vi "DispenseOnOff_Boolean.vi"(10 "Value":bool=TRUE, 11 "I-O in":refnum<class "Copy of I-O.lvclass">) -> (3 "I-O out":refnum<class "Copy of I-O.lvclass">)   [LabVIEW 2016]
uses:
  Copy of I-O.lvclass
panel:
  out "error out":errorcluster
  in  "error in (no error)":errorcluster
  # "Dispense On/Off"
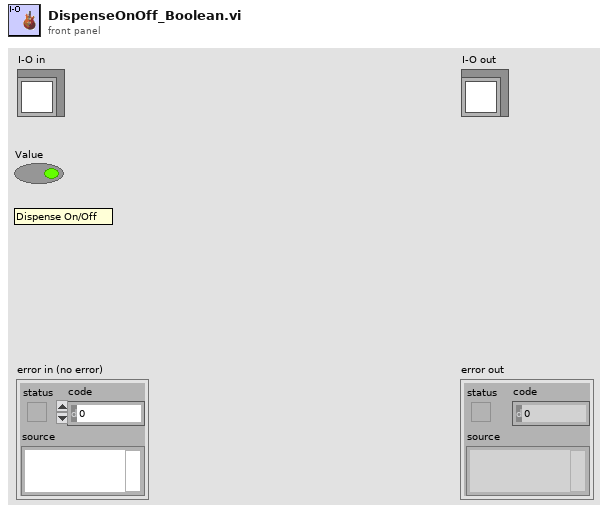
[diagram p1: front panel]
types:
  T1 = typedef "Copy of I-O.lvclass/Pin Map.ctl" = cluster{"Region Valves":i32[], "Extra Valves":dbl[][], "Tool Primary Valve":i32, "Tool Secondary Valve":i32, "Region Sensors":i32[], "Extra Sensors":dbl[][], "Tool Primary Sensor":dbl, "Tool Secondary Sensor":dbl, "Compression Sensor":dbl, "5V":i32, "NTU_Glue":dbl}
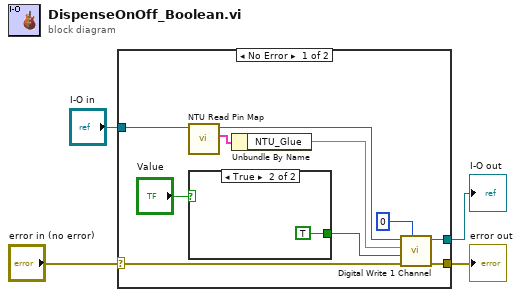
[diagram p0: block diagram]
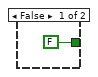
[diagram p2: hidden frame]
diagram:
  n1 = case shown="No Error" "error in (no error)" {
    selector: "error in (no error)" -> [w13 w18]
    tunnel: [w12 w18] -> w3
    tunnel: [w14 w17] -> w1
    tunnel: "I-O in" -> [w7 w17]
    frame No Error {
      n2 = call-dynamic "NTU Read Pin Map.vi"("I-O in"=w7) -> ("Pin Map"=w6:T1, "I-O out"=w5:refnum<class "Copy of I-O.lvclass">)  [unwired: 8 in, 1 out]
      n3 = case shown="True" "Value" {
        tunnel: [FALSE TRUE] -> w9
        frame False {
        }
        frame True {
        }
      }
      n4 = Unbundle By Name(w6) -> ("NTU_Glue"=w11:dbl)
      n5 = call-dynamic "Digital Write 1 Channel.vi"("DAQ Module"=0, "error constant"=w13, "Value"=w9, "Channel"=w11, "I-O.lvclass"=w5) -> ("error IO"=w12:errorcluster, "I-O.lvclass 2"=w14:refnum<class "Copy of I-O.lvclass">)  [unwired: 5 in]
    }
    frame Error {
    }
  }
  "error out" <- w3
  "I-O out" <- w1
